vi "Mappa AI DI PLC_2.vi"(0 "USCITE PLC":T1, 1 "MBit read":bool[](array[boolean]), 2 "MW read":dbl[](array[numeric]), 3 "M real read":dbl[](array[numeric]), 4 "Array DB bit":bool[](array[boolean]), 5 "DB WORD":dbl[](array[numeric]), 7 "DB REAL":dbl[](array[numeric])) -> (14 "STATO PLC":T4)   [LabVIEW 2019]
uses:
  STATO PLC 2.ctl
  Uscite PLC 2.ctl
  controls/statoAO_plc_2.ctl
  StatoDO_PLC_2.ctl
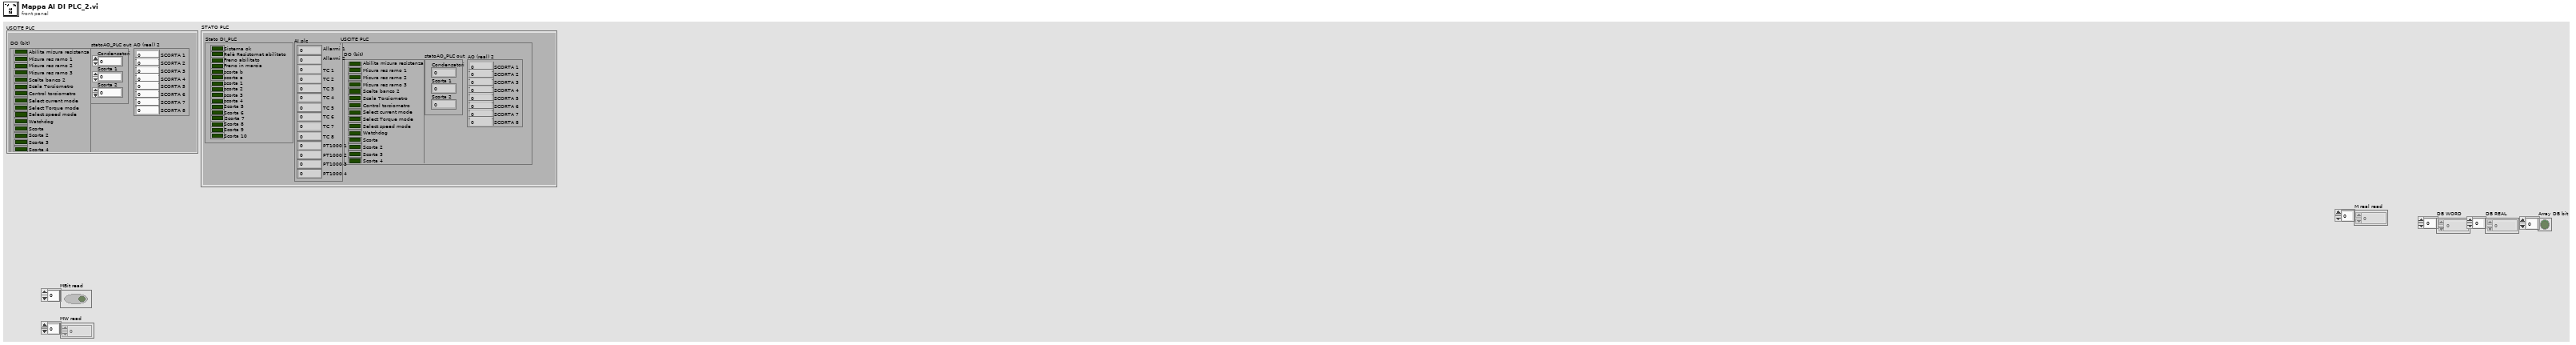
[diagram p1: front panel]
types:
  T1 = typedef "Uscite PLC 2.ctl" = cluster{"AO (real) 2":cluster{"SCORTA 1":dbl, "SCORTA 2":dbl, "SCORTA 3":dbl, "SCORTA 4":dbl, "SCORTA 5":dbl, "SCORTA 6":dbl, "SCORTA 7":dbl, "SCORTA 8":dbl}, "statoAO_PLC out":T2, "DO (bit)":T3}
  T2 = typedef "statoAO_plc_2.ctl" = cluster{"Condensatori":dbl, "Scorta 1":dbl, "Scorta 2":dbl}
  T3 = typedef "StatoDO_PLC_2.ctl" = cluster{"Relè misura resistomat":bool, "Misura res ramo 1":bool, "Misura res ramo 2":bool, "Misura res ramo 3":bool, "Scelta banco 2":bool, "Scala Torsiometro":bool, "Ctrl torsiometro":bool, "Select current mode":bool, "Select Torque mode":bool, "Select speed mode":bool, "Watchdog":bool, "Scorta":bool, "Scorta 2":bool, "Scorta 3":bool, "Scorta 4":bool, "Scorta 5":bool, "Bench selection":bool, "External alarm":bool, "Enable external program":bool, "Reset allarmi":bool, "Start":bool, "Stop":bool, "Block":bool, "Scorta 6":bool}
  T4 = typedef "STATO PLC 2.ctl" = cluster{"USCITE PLC":T1, "Stato DI_PLC":cluster{"Sistema ok":bool, "Relè Resistomat abilitato":bool, "Freno abilitato":bool, "Freno in marcia":bool, "scorta b":bool, "scorta a":bool, "scorta 1":bool, "scorta 2":bool, "scorta 3":bool, "scorta 4":bool, "Scorta 5":bool, "Scorta 6":bool, "Scorta 7":bool, "Scorta 8":bool, "Scorta 9":bool, "Scorta 10":bool}, "AI plc":cluster{"Allarmi 1":dbl, "Allarmi 2":dbl, "TC 1":dbl, "TC 2":dbl, "TC 3":dbl, "TC 4":dbl, "TC 5":dbl, "TC 6":dbl, "TC 7":dbl, "TC 8":dbl, "PT1000 1":dbl, "PT1000 2":dbl, "PT1000 3":dbl, "PT1000 4":dbl}}
  T5 = cluster{"MBit read[0]":bool, "MBit read[1]":bool, "MBit read[2]":bool, "MBit read[3]":bool, "MBit read[4]":bool, "MBit read[5]":bool, "MBit read[6]":bool, "MBit read[7]":bool, "MBit read[8]":bool, "MBit read[9]":bool, "MBit read[10]":bool, "MBit read[11]":bool, "MBit read[12]":bool, "MBit read[13]":bool, "MBit read[14]":bool, "MBit read[15]":bool}
  T6 = cluster{"MW read[0]":dbl, "MW read[1]":dbl, "MW read[2]":dbl, "MW read[3]":dbl, "MW read[4]":dbl, "MW read[5]":dbl, "MW read[6]":dbl, "MW read[7]":dbl, "MW read[8]":dbl, "MW read[9]":dbl, "MW read[10]":dbl, "MW read[11]":dbl, "MW read[12]":dbl, "MW read[13]":dbl}
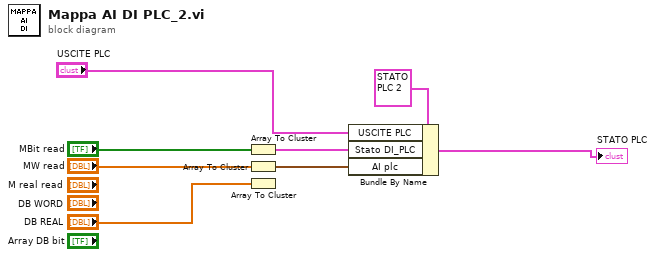
[diagram p0: block diagram]
diagram:
  n1 = Array To Cluster(array="MBit read") -> (cluster=w4:T5)
  n2 = Array To Cluster(array="MW read") -> (cluster=w2:T6)
  n3 = Array To Cluster(array="DB REAL") -> ()  [unwired: 1 out]
  n4 = Bundle By Name(cluster=T4 {"USCITE PLC"={"AO (real) 2"={"SCORTA 1"=0.0, "SCORTA 2"=0.0, "SCORTA 3"=0.0, "SCORTA 4"=0.0, "SCORTA 5"=0.0, "SCORTA 6"=0.0, "SCORTA 7"=0.0, "SCORTA 8"=0.0}, "statoAO_PLC out"={"Condensatori"=0.0, "Scorta 1"=0.0, "Scorta 2"=0.0}, "DO (bit)"={"Relè misura resistomat"=FALSE, "Misura res ramo 1"=FALSE, "Misura res ramo 2"=FALSE, "Misura res ramo 3"=FALSE, "Scelta banco 2"=FALSE, "Scala Torsiometro"=FALSE, "Ctrl torsiometro"=FALSE, "Select current mode"=FALSE, "Select Torque mode"=FALSE, "Select speed mode"=FALSE, "Watchdog"=FALSE, "Scorta"=FALSE, "Scorta 2"=FALSE, "Scorta 3"=FALSE, "Scorta 4"=FALSE, "Scorta 5"=FALSE, "Bench selection"=FALSE, "External alarm"=FALSE, "Enable external program"=FALSE, "Reset allarmi"=FALSE, "Start"=FALSE, "Stop"=FALSE, "Block"=FALSE, "Scorta 6"=FALSE}}, "Stato DI_PLC"={"Sistema ok"=FALSE, "Relè Resistomat abilitato"=FALSE, "Freno abilitato"=FALSE, "Freno in marcia"=FALSE, "scorta b"=FALSE, "scorta a"=FALSE, "scorta 1"=FALSE, "scorta 2"=FALSE, "scorta 3"=FALSE, "scorta 4"=FALSE, "Scorta 5"=FALSE, "Scorta 6"=FALSE, "Scorta 7"=FALSE, "Scorta 8"=FALSE, "Scorta 9"=FALSE, "Scorta 10"=FALSE}, "AI plc"={"Allarmi 1"=0.0, "Allarmi 2"=0.0, "TC 1"=0.0, "TC 2"=0.0, "TC 3"=0.0, "TC 4"=0.0, "TC 5"=0.0, "TC 6"=0.0, "TC 7"=0.0, "TC 8"=0.0, "PT1000 1"=0.0, "PT1000 2"=0.0, "PT1000 3"=0.0, "PT1000 4"=0.0}} ("STATO PLC"), "USCITE PLC"="USCITE PLC", "Stato DI_PLC"=w4, "AI plc"=w2) -> (→"STATO PLC":T4)
